vi "Read Setup.vi"(8 "error in":errorcluster, 11 "File Path in":path) -> (0 "error out":errorcluster, 2 "Setup Data":T1={"DataBase Data"={"Api Token"="", "Organization"="", "url"="", "Organization ID"=""}, "Query - csv"="", "Bucket"="", "Measurement"="", "Timestamp precision"=enum."Seconds", "Tags"=[{"Key"="host1", "Value"="myPC"}, {"Key"="host2", "Value"="X-Server"}]}, 3 "File Path out":path)   [LabVIEW 2020]
doc: "Reads all settings for the test application from the setup file"
uses:
  Setup Data.ctl
  InfluxDB v2 Client/Client/DataBase Data.ctl
  InfluxDB v2 Client/Client/Write Precision.ctl
  InfluxDB v2 Client/Data Point/Tag.ctl
  <vilib>/Utility/xml.llb/Read From XML File(string).vi
  InfluxDB v2 Client/InfluxDB v2 Client.lvlib
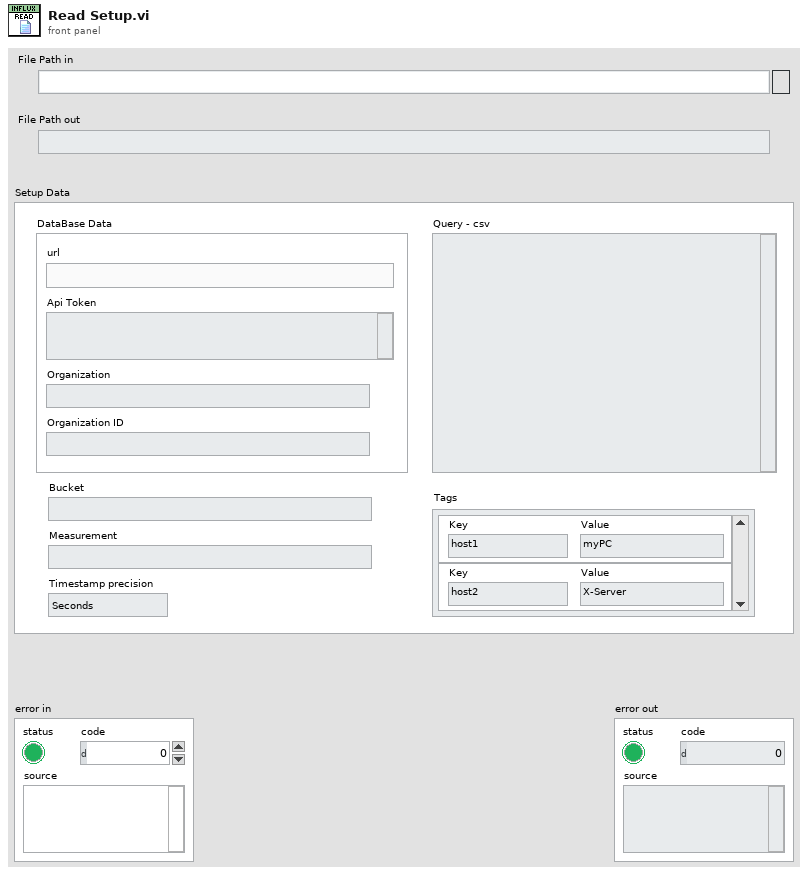
[diagram p1: front panel]
types:
  T1 = typedef "Setup Data.ctl" = cluster{"DataBase Data":T2, "Query - csv":string, "Bucket":string, "Measurement":string, "Timestamp precision":T3, "Tags":T4[]}
  T2 = typedef "InfluxDB v2 Client.lvlib/DataBase Data.ctl" = cluster{"Api Token":string, "Organization":string, "url":string, "Organization ID":string}
  T3 = typedef "InfluxDB v2 Client.lvlib/Write Precision.ctl" = enum16{"Nanoseconds", "Microseconds", "Milliseconds", "Seconds"}
  T4 = typedef "InfluxDB v2 Client.lvlib/Tag.ctl" = cluster{"Key":string, "Value":string}
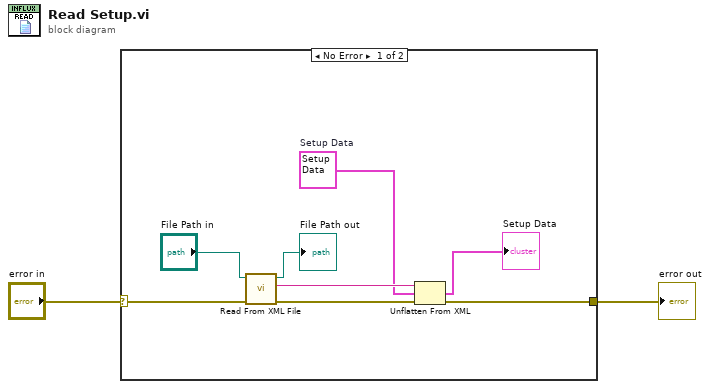
[diagram p0: block diagram]
diagram:
  n1 = case shown="No Error" "error in" {
    selector: "error in" -> [w10 w11]
    tunnel: [w6 w11] -> w1
    frame No Error {
      w3 = T1 {"DataBase Data"={"Api Token"="", "Organization"="", "url"="", "Organization ID"=""}, "Query - csv"="", "Bucket"="", "Measurement"="", "Timestamp precision"=enum."Seconds", "Tags"=[{"Key"="host1", "Value"="myPC"}, {"Key"="host2", "Value"="X-Server"}]}  # Setup Data
      n2 = call-poly <vilib>:"Read From XML File.vi"("error in (no error)"=w10, "XML File Path"="File Path in") -> ("error out"=w8:errorcluster, "XML Elements"=w7:string, "XML File Path(duplicate)"=→"File Path out":path)  [unwired: 7 in]
      n3 = Unflatten From XML(xml string=w7, type=w3, error in (no error)=w8) -> (value=→"Setup Data":T1, error out=w6:errorcluster)
    }
    frame Error {
    }
  }
  "error out" <- w1
